vi "Register Chart.vi"(8 "error in (no error)":errorcluster, 10 "Chart Registration":T1, 11 "Historian Charting Manager in":refnum<class "Historian Charting Manager.lvclass">) -> (0 "error out":errorcluster, 3 "Historian Charting Manager out":refnum<class "Historian Charting Manager.lvclass">)   [LabVIEW 2020, in "VolatusGUI.lvlib" / "Historian Charting Manager.lvclass"]
uses:
  Historian Charting Manager.lvclass
  Historian Charting Manager.lvclass/Historian Charting Manager.ctl
  Scale.ctl
  Plot Config.ctl
  X-Axis Type.ctl
  Plot Group Config.ctl
  Select Plot Group Data.ctl
  Chart Registration.ctl
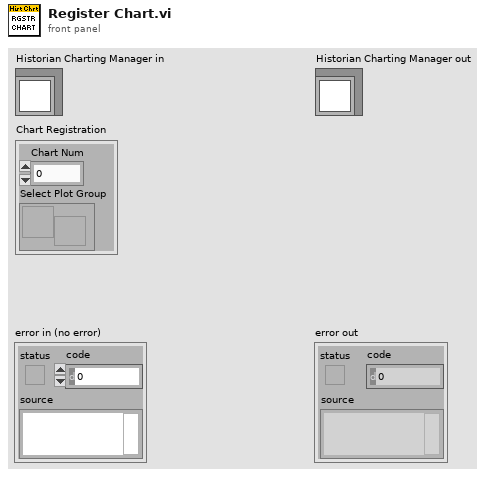
[diagram p1: front panel]
types:
  T1 = typedef "VolatusGUI.lvlib/Historian Charting Manager.lvclass/Chart Registration.ctl" = cluster{"Chart Num":i32, "Select Plot Group":refnum<user-event>}
  T2 = typedef "VolatusGUI.lvlib/Historian Charting Manager.lvclass/Select Plot Group Data.ctl" = cluster{"Chart Num":i32, "Plots Config":T3}
  T3 = typedef "VolatusGUI.lvlib/Historian Charting Manager.lvclass/Plot Group Config.ctl" = cluster{"Name":string, "X-Axis Type":T4, "X-Axis Channel":string, "Plots":T5[], "Lock Now":bool, "Time":string}
  T4 = typedef "VolatusGUI.lvlib/Historian Charting Manager.lvclass/X-Axis Type.ctl" = enum16{"Time", "Channel"}
  T5 = typedef "VolatusGUI.lvlib/Historian Charting Manager.lvclass/Plot Config.ctl" = cluster{"Channel":string, "Visible":bool, "Color":u32, "Scale":T6}
  T6 = typedef "VolatusGUI.lvlib/Historian Charting Manager.lvclass/Scale.ctl" = enum16{"Left", "Right"}
  T7 = typedef "VolatusGUI.lvlib/Historian Charting Manager.lvclass/Chart Info.ctl" = cluster{"PluginGUI":refnum<class "MessageQ.lvclass">, "Select Plot Group":refnum<user-event>}
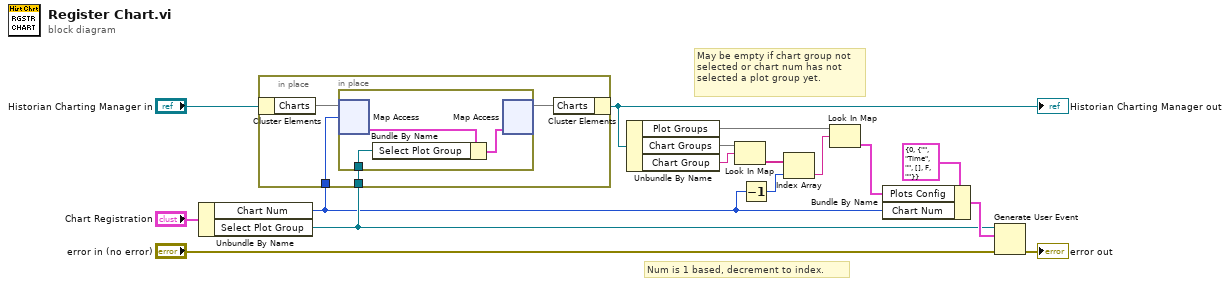
[diagram p0: block diagram]
diagram:
  # "May be empty if chart group not selected or chart num has not selected a plot group yet."
  # "Num is 1 based, decrement to index."
  n1 = Unbundle By Name("Chart Registration") -> ("Chart Num"=w3:i32, "Select Plot Group"=w5:refnum<user-event>)
  n2 = in-place {
    in-place-border: w3 -> [w19]
    in-place-border: w5 -> [w18]
    n3 = in-place-cluster #1("Historian Charting Manager in") -> ("Charts"=w20:map{i32, T7})
    n4 = in-place {
      in-place-border: w18 -> [w22]
      n5 = in-place-map #2(w20, w19) -> (w23:T7)  [unwired: 1 in, 1 out]
      n6 = Bundle By Name(cluster=w23, "Select Plot Group"=w22) -> (w21:T7)
      n7 = in-place-map #2(w21) -> (w17:map{i32, T7})  [unwired: 1 in, 2 out]
    }
    n8 = in-place-cluster #1("Charts"=w17) -> (w1:refnum<class "Historian Charting Manager.lvclass">)
  }
  "Historian Charting Manager out" <- w1
  n9 = Unbundle By Name(w1) -> ("Plot Groups"=w11:map{string, T3}, "Chart Groups"=w16:map{string, string[]}, "Chart Group"=w15:string)
  n10 = Look In Map(map=w16, key=w15) -> (value=w14:string[])  [unwired: 1 in, 1 out]
  n11 = Decrement(x=w3) -> (x-1=w4:i32)
  n12 = Index Array(array=w14, index=w4) -> (element=w10:string)
  n13 = Look In Map(map=w11, key=w10) -> (value=w9:T3)  [unwired: 1 in, 1 out]
  n14 = Bundle By Name(cluster=T2 {"Chart Num"=0, "Plots Config"={"Name"="", "X-Axis Type"=enum."Time", "X-Axis Channel"="", "Plots"=[], "Lock Now"=FALSE, "Time"=""}} ("event data"), "Plots Config"=w9, "Chart Num"=w3) -> (w12:T2)
  n15 = Generate User Event(user event=w5, event data cluster=w12, error in="error in (no error)") -> (error out=→"error out":errorcluster)  [unwired: 1 in, 1 out]
